vi "Index By RH.vi"(1 "Relative Humidity":dbl) -> (0 "RH Index":dbl)   [LabVIEW 2020]
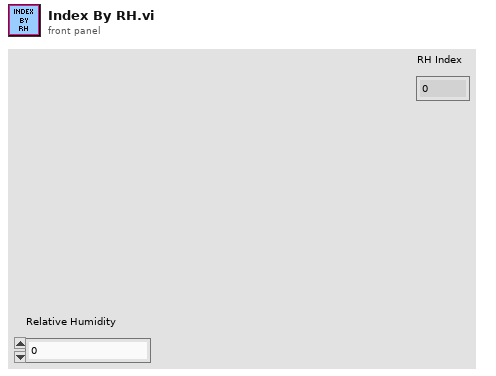
[diagram p1: front panel]
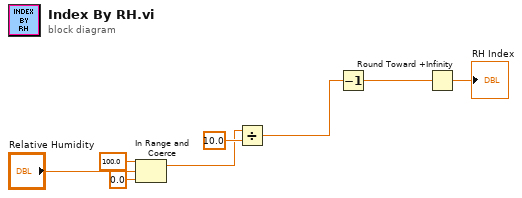
[diagram p0: block diagram]
diagram:
  n1 = In Range and Coerce(upper limit=100.0, x="Relative Humidity", lower limit=0.0) -> (coerced(x)=w5:dbl)  [unwired: 1 out]
  n2 = Divide(x=w5, y=10.0) -> (x/y=w2:dbl)
  n3 = Decrement(x=w2) -> (x-1=w1:dbl)
  n4 = Round Toward +Infinity(x=w1) -> (ceil(x): smallest int >= x=→"RH Index":dbl)
